vi "Open Waveform Streaming Manager Reference.vi"(8 "error in (no error)":errorcluster, 11 "Gateway IP Address (\"\": localhost)":string) -> (0 "error out":errorcluster, 3 "WaveformStreaming":T1)   [LabVIEW 2020, in "NI_VS Waveform Streaming Interface.lvlib"]
doc: "Opens a reference to the waveform-stream manager on the VeriStand Gateway. You must open a reference before you register to receive waveform data and start streaming waveforms from the VeriStand Gateway."
uses:
  <vilib>/NI VeriStand/Execution/WaveformStreaming/NI_VS Waveform Streaming Interface.lvlib
  <vilib>/NI VeriStand/Execution/WaveformStreaming/WaveformStreamingAPI.ctl
  NationalInstruments.VeriStand.ClientAPI
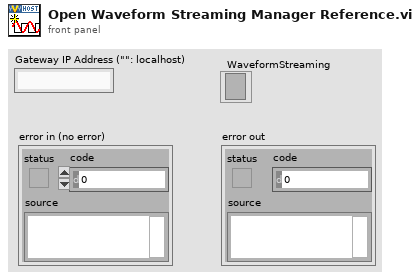
[diagram p1: front panel]
types:
  T1 = typedef "NI_VS Waveform Streaming Interface.lvlib/WaveformStreamingAPI.ctl" = refnum<k24>
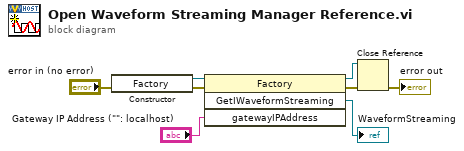
[diagram p0: block diagram]
diagram:
  n1 = constructor class="Factory"(error in="error in (no error)") -> (reference out=w7:refnum<k24>, error out=w8:errorcluster)  [unwired: 2 in, 1 out]
  n2 = invoke class="Factory" method="GetIWaveformStreaming"(reference=w7, error in=w8, "gatewayIPAddress"="Gateway IP Address (\"\": localhost)") -> (reference out=w5:refnum<k24>, error out=w6:errorcluster, "GetIWaveformStreaming"=→"WaveformStreaming":refnum<k24>)  [unwired: 1 in, 1 out]
  n3 = Close Reference(reference=w5, error in (no error)=w6) -> (error out=→"error out":errorcluster)
